vi "REPL_Clean.vi"(11 "Code in":string) -> (3 "Code cleaned":string)   [LabVIEW 2020]
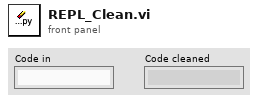
[diagram p1: front panel]
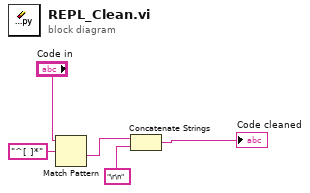
[diagram p0: block diagram]
diagram:
  n1 = Match Pattern(string="Code in", regular expression="^[ ]*") -> (after substring=w5:string)  [unwired: 1 in, 3 out]
  n2 = Concatenate Strings(w5, "\r\n" ("write buffer")) -> (→"Code cleaned":string)
